vi "Get images from queue.vi"(8 "error in":errorcluster) -> (0 "error out":errorcluster)   [LabVIEW 2012]
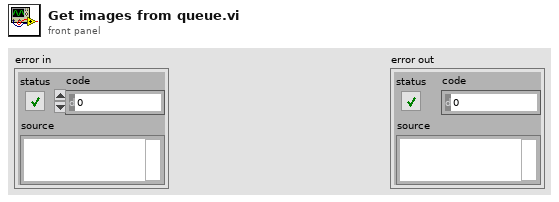
[diagram p1: front panel]
types:
  T1 = typedef "Image Type" = u32
  T2 = cluster{"Array uint 16":u16[][], "setting.File Path":path}
  T3 = typedef "IMAQ Image.ctl" = refnum<image>
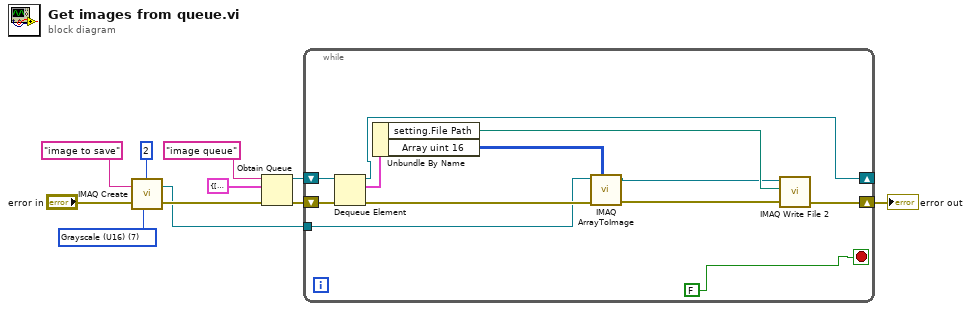
[diagram p0: block diagram]
diagram:
  w1 = T1 7 items=["Grayscale (U8)", "Grayscale (I16)", "Grayscale (SGL)", "Complex (CSG)", "RGB (U32)", "HSL (U32)", "RGB (U64)", "Grayscale (U16)"] ("Image Type")
  n1 = call "IMAQ Create"("Border Size"=2, "Image Name"="image to save", "Image Type"=w1, "error in (no error)"="error in") -> ("New Image"=w2:T3, "error out"=w3:errorcluster)  [unwired: 1 in]
  n2 = Obtain Queue(name (unnamed)="image queue", element data type=T2 {"Array uint 16"=[], "setting.File Path"=path ""} ("queue elemet type"), error in (no error)=w3) -> (queue out=w8:refnum<queue>, error out=w10:errorcluster)  [unwired: 2 in, 1 out]
  n3 = while {
    shift-right: [w16] -> w11
    shift-left: w10 -> [w23]
    tunnel: w2 -> [w19]
    shift-right: [w13] -> _
    shift-left: w8 -> [w22]
    stop <- FALSE stop-if-true
    n4 = Dequeue Element(queue=w22, error in (no error)=w23) -> (queue out=w13:refnum<queue>, element=w21:T2, error out=w20:errorcluster)  [unwired: 1 in, 1 out]
    n5 = Unbundle By Name(w21) -> ("setting.File Path"=w17:path, "Array uint 16"=w18:u16[][])
    n6 = call "IMAQ ArrayToImage"("Image Pixels (U16)"=w18, "error in (no error)"=w20, "Image"=w19) -> ("error out"=w14:errorcluster, "Image Out"=w15:T3)  [unwired: 7 in]
    n7 = call-poly "IMAQ Write File 2"("error in (no error)"=w14, "File Path"=w17, "Image"=w15) -> ("error out"=w16:errorcluster)  [unwired: 7 in, 1 out]
  }
  "error out" <- w11
